vi "Init.vi"(8 "error in (no error)":errorcluster, 9 "ICameraTesting":refnum<class "ICameraTesting.lvclass">, 10 "CameraInfo":T1, 11 "CameraTestingProxy":refnum<class "CameraTestingProxyAPI.lvclass">) -> (0 "error out":errorcluster, 3 "CameraTestingProxy":refnum<class "CameraTestingProxyAPI.lvclass">)   [LabVIEW 2020, in "CameraTestingProxy.lvlib" / "CameraTestingProxyAPI.lvclass"]
uses:
  CameraTestingProxyAPI.lvclass
  CameraTestingApp/ICameraTesting/TypeDef/CameraInfo.ctl
  Camera/ICamera/ICamera/ICamera.lvclass
  CameraTestingApp/ICameraTesting/ICameraTesting/ICameraTesting.lvclass
  CameraTestingENI/Community/TypeDef/RequestEventList.ctl
  ICameraTestingProxy/TypeDef/VideoFrameData.ctl
  CameraTestingProxyAPI.lvclass/CameraTestingProxyAPI.ctl
  CameraTestingENI/CameraTestingENI.lvclass
  ICameraTestingProxy/TypeDef/ICameraTestingProxy_typedef.lvlib
  CameraTestingApp/ICameraTesting/TypeDef/ICameraTesting_typedef.lvlib
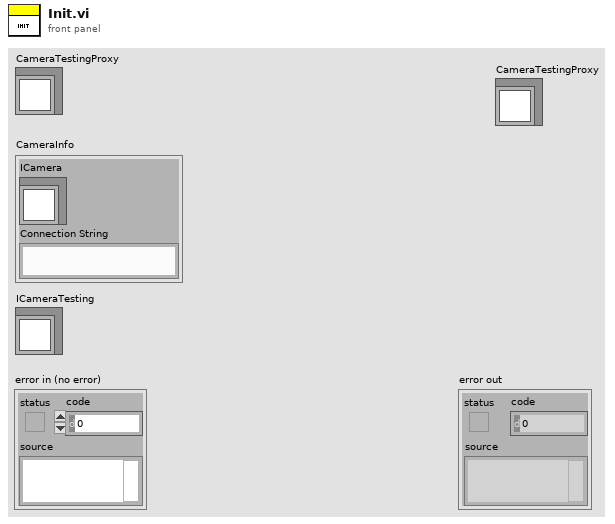
[diagram p1: front panel]
types:
  T1 = typedef "ICameraTesting_typedef.lvlib/CameraInfo.ctl" = cluster{"ICamera ":refnum<class "ICamera.lvclass">, "Connection String":string}
  T2 = typedef "ICameraTestingProxy_typedef.lvlib/VideoFrameData.ctl" = cluster{"image depth":i32, "Data[]":u8[], "Bounds":cluster{"Height":i16, "Width":i16}}
  T3 = typedef "CameraTestingProxy.lvlib/CameraTestingENI.lvclass/RequestEventList.ctl" = cluster{"ConnectCmd":refnum<user-event>, "PlayCmd":refnum<user-event>, "SnapShoot":refnum<user-event>, "GetResolution":refnum<user-event>, "GetImageType":refnum<user-event>, "GetFrameRate":refnum<user-event>, "AcqVideoOptCodes":refnum<user-event>, "Quit":refnum<user-event>, "SetResolution":refnum<user-event>, "SetImageType":refnum<user-event>, "SetFrameRate":refnum<user-event>}
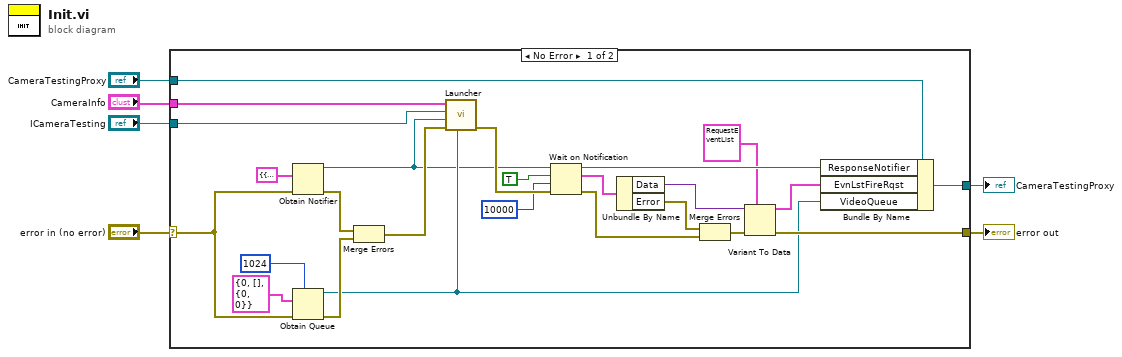
[diagram p0: block diagram]
diagram:
  n1 = case shown="No Error" "error in (no error)" {
    selector: "error in (no error)" -> [w15 w33]
    tunnel: [w31 w33] -> w6
    tunnel: [w29 w32] -> w5
    tunnel: "CameraTestingProxy" -> [w11 w32]
    tunnel: "CameraInfo" -> [w8 _]
    tunnel: "ICameraTesting" -> [w7 _]
    frame No Error {
      n2 = Obtain Notifier(notification data type=cluster{"Error":errorcluster, "Data":variant} {"Error"={"status"=FALSE, "code"=0, "source"=""}, "Data"=variant}, error in (no error)=w15) -> (notifier out=w9:refnum<notifier>, error out=w14:errorcluster)  [unwired: 2 in, 1 out]
      n3 = Obtain Queue(max queue size (-1, unlimited)=1024, element data type=T2 {"image depth"=0, "Data[]"=[], "Bounds"={"Height"=0, "Width"=0}} ("VideoFrameData"), error in (no error)=w15) -> (queue out=w10:refnum<queue>, error out=w13:errorcluster)  [unwired: 2 in, 1 out]
      n4 = Merge Errors(w14, w13) -> (w12:errorcluster)
      n5 = call "Launcher.vi"("VideoQueue"=w10, "error in (no error)"=w12, "ResponseNotifier"=w9, "ICameraTesting"=w7, "CameraInfo"=w8) -> ("error out"=w24:errorcluster)  [unwired: 6 in]
      n6 = Wait on Notification(notifier=w9, ignore previous (F)=TRUE, timeout in ms (-1)=10000, error in (no error)=w24) -> (notifier out=w25:refnum<notifier>, notification=w22:cluster{"Error":errorcluster, "Data":variant}, error out=w21:errorcluster)  [unwired: 1 out]
      n7 = Unbundle By Name(w22) -> ("Data"=w18:variant, "Error"=w20:errorcluster)
      n8 = Merge Errors(w20, w21) -> (w19:errorcluster)
      n9 = Variant To Data(error in=w19, type=T3 {"ConnectCmd"=refnum, "PlayCmd"=refnum, "SnapShoot"=refnum, "GetResolution"=refnum, "GetImageType"=refnum, "GetFrameRate"=refnum, "AcqVideoOptCodes"=refnum, "Quit"=refnum, "SetResolution"=refnum, "SetImageType"=refnum, "SetFrameRate"=refnum} ("EvnLstFireRqst"), Variant=w18) -> (data=w28:T3, error out=w31:errorcluster)
      n10 = Bundle By Name(cluster=w11, "ResponseNotifier"=w25, "EvnLstFireRqst"=w28, "VideoQueue"=w10) -> (w29:refnum<class "CameraTestingProxyAPI.lvclass">)
    }
    frame Error {
    }
  }
  "error out" <- w6
  "CameraTestingProxy" <- w5
